vi "max30102Chart_Plot_step1.vi"() -> ()   [LabVIEW 2014]
doc: "Use this template to build a producer/consumer design pattern. Use this template when you need to execute a process, such as data analysis, when a data source, such as a triggered acquisition, produces data at an uneven rate and you need to execute the process when the data becomes available.\n------------------------------------\nAuther: Koji Ohashi\nCopyright (c) 2020 Japan LabVIEW Users Group, Volunteer members.\nThis VI is released under the MIT License.\nhttp://opensource.org/licenses/mit-license.php\n------------------------------------"
uses:
  <vilib>/Instr/_visa.llb/VISA Configure Serial Port (Instr).vi
panel:
  out "Waveform Chart":i32(graph)
  in  "Read Count":u32=1000
  in  "Termination Character":u8=10 format="%.0x"
  in  "VISA resource name":refnum<visa-resource-name>="COM1"
  in  "Serial Settings":T1={"baud rate"=9600, "data bits"=8, "parity"=enum."None", "stop bits"=10, "flow control"=0} {"flow control" items=["None"=0, "XON/XOFF"=1, "RTS/CTS"=2, "DTR/DSR"=4]; "stop bits" items=["1.0"=10, "1.5"=15, "2.0"=20]; "data bits" min=5 max=8 step=1; "baud rate" items=["75"=75, "110"=110, "134"=134, "150"=150, "300"=300, "600"=600, "1200"=1200, "1800"=1800, "2400"=2400, "4800"=4800, "7200"=7200, "9600"=9600, "14400"=14400, "19200"=19200, "28800"=28800, "38400"=38400, "56000"=56000, "57600"=57600, "115200"=115200, "128000"=128000, "230400"=230400]}
  in  "End Read on Termination Character?":bool=TRUE
  in  "stop":bool
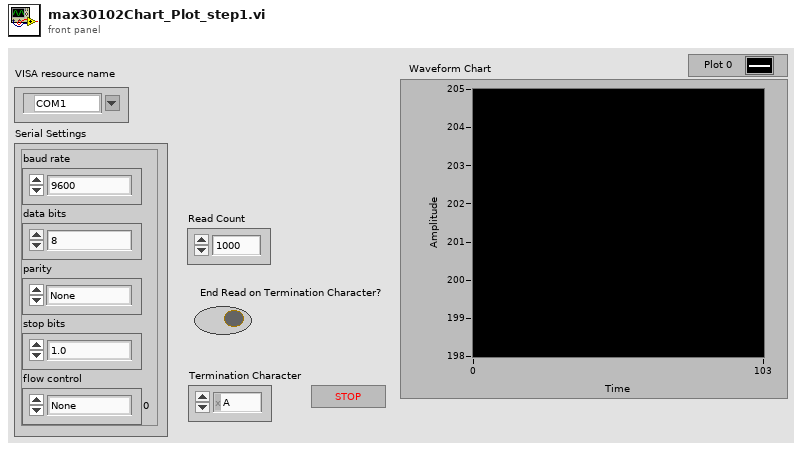
[diagram p1: front panel]
types:
  T1 = cluster{"baud rate":u32, "data bits":u16, "parity":enum16{"None", "Odd", "Even", "Mark", "Space"}, "stop bits":u16, "flow control":u16}
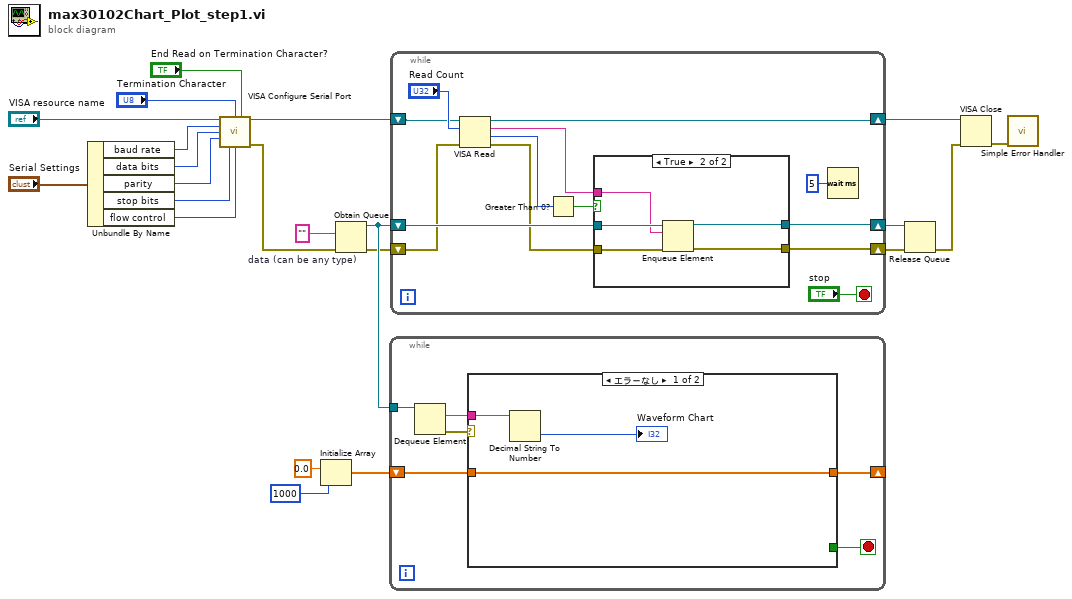
[diagram p0: block diagram]
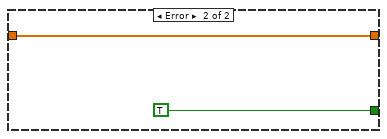
[diagram p2: hidden frame]
diagram:
  w18 = ""  # data (can be any type)
  n1 = Unbundle By Name("Serial Settings") -> ("baud rate"=w13:u32, "data bits"=w14:u16, "parity"=w15:enum16{"None", "Odd", "Even", "Mark", "Space"}, "stop bits"=w16:u16, "flow control"=w10:u16)
  n2 = call-poly "VISA Configure Serial Port"("VISA resource name"="VISA resource name", "termination char\n(0xA = '\\n' = LF)"="Termination Character", "Enable Termination\nChar (T)"="End Read on Termination Character?", "baud rate (9600)"=w13, "data bits (8)"=w14, "parity (0:none)"=w15, "stop bits (10: 1 bit)"=w16, "flow control (0:none)"=w10) -> ("VISA resource name out"=w8:refnum<visa-resource-name>, "error out"=w5:errorcluster)  [unwired: 2 in, 4 out]
  n3 = Initialize Array(0.0 ("element"), 1000 ("dimension size")) -> (w1:dbl[])
  n4 = Obtain Queue(element data type=w18, error in (no error)=w5) -> (queue out=w22:refnum<queue>, error out=w21:errorcluster)  [unwired: 3 in, 1 out]
  n5 = while {
    tunnel: w22 -> [w28]
    shift-right: [w23] -> _
    shift-left: w1 -> [w24]
    stop <- w25 stop-if-true
    n6 = Dequeue Element(queue=w28) -> (element=w26:string, error out=w27:errorcluster)  [unwired: 2 in, 2 out]
    n7 = case shown="エラーなし" w27 {
      tunnel: w26 -> [w31 _]
      tunnel: [_ TRUE] -> w25
      tunnel: w24 -> [w29 w32]
      tunnel: [w29 w32] -> w23
      frame No Error {
        n8 = Decimal String To Number(string=w31) -> (number=→"Waveform Chart":i32)  [unwired: 2 in, 1 out]
      }
      frame Error {
      }
    }
  }
  n9 = while {
    shift-right: [w43] -> w19
    shift-left: w21 -> [w36]
    shift-right: [w44] -> w20
    shift-left: w22 -> [w45]
    shift-right: [w40] -> w6
    shift-left: w8 -> [w34]
    stop <- "stop" stop-if-true
    n10 = VISA Read(VISA resource name=w34, byte count="Read Count", error in (no error)=w36) -> (VISA resource name out=w40:refnum<visa-resource-name>, read buffer=w37:string, return count=w39:u32, error out=w35:errorcluster)
    n11 = Greater Than 0?(x=w39) -> (x > 0?=w38:bool)
    n12 = case shown="TRUE" w38 {
      tunnel: w45 -> [w48 w53]
      tunnel: [w48 w52] -> w44
      tunnel: w35 -> [w47 w51]
      tunnel: [w47 w50] -> w43
      tunnel: w37 -> [_ w49]
      frame False {
      }
      frame True {
        n13 = Enqueue Element(queue=w53, element=w49, error in (no error)=w51) -> (queue out=w52:refnum<queue>, error out=w50:errorcluster)  [unwired: 1 in, 1 out]
      }
    }
    n14 = Wait (ms)(milliseconds to wait=u32 5) -> ()  [unwired: 1 out]
  }
  n15 = Release Queue(queue=w20, error in (no error)=w19) -> (error out=w4:errorcluster)  [unwired: 1 in, 2 out]
  n16 = VISA Close(VISA resource name=w6, error in (no error)=w4) -> (error out=w7:errorcluster)
  n17 = call <vilib>:"Simple Error Handler.vi"("error in (no error)"=w7) -> ()  [unwired: 1 in, 8 out]
